vi "tsdiag_can_security_access_send_key.vi"(6 "ATimeoutMS":i32, 8 "AKeyValue":u8[](array[numeric]), 9 "ALevel":i32, 10 "ADiagModuleIndex":i32, 11 "路径输入":path) -> (2 "返回类型":i32, 3 "路径输出":path)   [LabVIEW 2019]
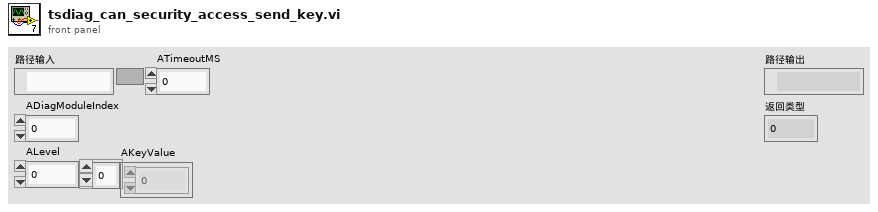
[diagram p1: front panel]
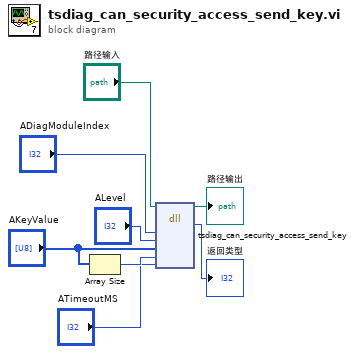
[diagram p0: block diagram]
diagram:
  n1 = Array Size(array="AKeyValue") -> (size(s)=w3:i32)
  n2 = dll-call lib="C:/Users/XYY/Desktop/LabView Demo/TSCAN_LB2018_V1.4_20220309/Config/TSMaster.dll" fn="tsdiag_can_security_access_send_key"(path in="路径输入", "ADiagModuleIndex"="ADiagModuleIndex", "ALevel"="ALevel", "AKeyValue"="AKeyValue", "AKeySize"=w3, "ATimeoutMS"="ATimeoutMS") -> (path out=→"路径输出":path, "返回类型"=→"返回类型":i32)  [unwired: 7 in, 1 out]
